vi "Write Allow Multiple Names.vi"(8 "error in (no error)":errorcluster, 10 "AllowMultNames":bool, 11 "DAQChannelName.lvclass in":refnum<class "DAQChannelName.lvclass">) -> (0 "error out":errorcluster, 3 "DAQChannelName.lvclass out":refnum<class "DAQChannelName.lvclass">)   [LabVIEW 2015, in "DAQChannelName.lvclass"]
uses:
  DAQChannelName.lvclass
  DAQChannelName.lvclass/DAQChannelName.ctl
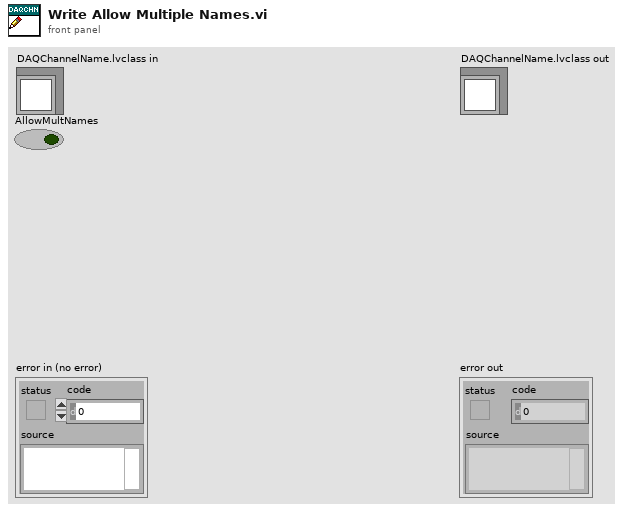
[diagram p1: front panel]
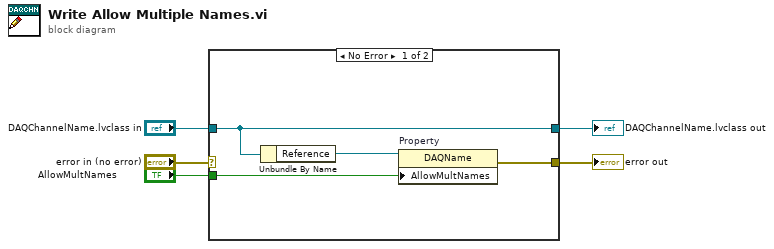
[diagram p0: block diagram]
diagram:
  n1 = case shown="No Error" "error in (no error)" {
    selector: "error in (no error)" -> [_ w11]
    tunnel: [w9 w11] -> w4
    tunnel: [w7 w10] -> w2
    tunnel: "DAQChannelName.lvclass in" -> [w7 w10]
    tunnel: "AllowMultNames" -> [w8 _]
    frame No Error {
      n2 = Unbundle By Name(w7) -> ("Reference"=w6:refnum<vi>)
      n3 = property on="Property" class="DAQName"(reference=w6, "AllowMultNames"=w8) -> (error out=w9:errorcluster)  [unwired: 1 in, 1 out]
    }
    frame Error {
    }
  }
  "error out" <- w4
  "DAQChannelName.lvclass out" <- w2
